vi "Walk Button.vi"() -> (0 "element":bool)   [LabVIEW 2012]
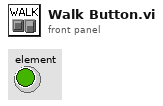
[diagram p1: front panel]
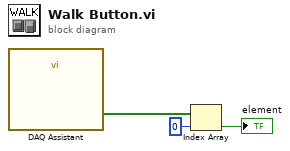
[diagram p0: block diagram]
diagram:
  n1 = call "DAQ Assistant"() -> ("data"=w3:bool[])  [unwired: 17 in, 2 out]
  n2 = Index Array(array=w3, index=0) -> (element=→"element":bool)
